vi "Bold Format Title.vi"(11 "Message Log in":refnum<class "Message Log.lvclass">) -> ()   [LabVIEW 2017, in "Message Log.lvclass"]
uses:
  Message Log.lvclass
  Message Log.lvclass/Message Log.ctl
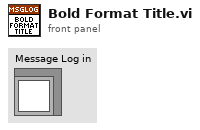
[diagram p1: front panel]
types:
  T1 = typedef "Message Log ID.ctl" = cluster{"Head Worker ID":string, "IP Address":string}
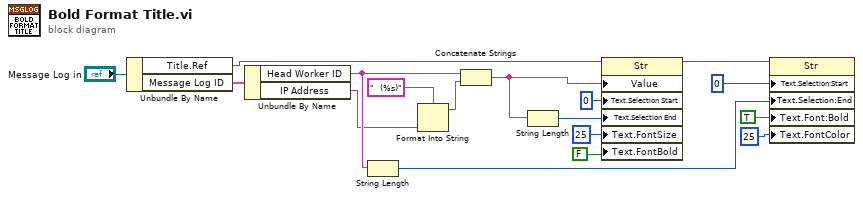
[diagram p0: block diagram]
diagram:
  n1 = Unbundle By Name("Message Log in") -> ("Title.Ref"=w15:refnum<vi>, "Message Log ID"=w16:T1)
  n2 = Unbundle By Name(w16) -> ("Head Worker ID"=w11:string, "IP Address"=w10:string)
  n3 = String Length(string=w11) -> (length=w8:i32)
  n4 = Format Into String(format string="  (%s)", w10) -> (resulting string=w9:string)  [unwired: 2 in, 1 out]
  n5 = Concatenate Strings(w11, w9) -> (w2:string)
  n6 = String Length(string=w2) -> (length=w1:i32)
  n7 = property class="Str"(reference=w15, "Value"=w2, "Text.Selection Start"=u32 0 ("Text.Selection:Start"), "Text.Selection End"=w1, "Text.FontSize"=u32 25 ("Text.Font:Size"), "Text.FontBold"=FALSE ("Text.Font:Bold")) -> (reference out=w14:refnum<vi>)  [unwired: 1 in, 1 out]
  n8 = property on="Property Node" class="Str"(reference=w14, "Text.Selection:Start"=u32 0, "Text.Selection:End"=w8, "Text.Font:Bold"=TRUE, "Text.FontColor"=u32 25 ("Text.Font:Color")) -> ()  [unwired: 1 in, 2 out]
